vi "LEBITVacuum.ProcCases.vi"(0 "i ref in":refnum<vi>, 1 "selector":string, 2 "Data":T1, 3 "call cluster":T2={"Object"="", "Selector"="", "CallType"=enum."synchronous", "Async Object"="", "Async Selector"="", "Data Descriptor"="", "Data"=[], "Error #"=0, "Expire"=0}, 5 "error in (no error)":errorcluster) -> (14 "i ref out":refnum<vi>, 17 "answer cluster":T2={"Object"="", "Selector"="", "CallType"=enum."synchronous", "Async Object"="", "Async Selector"="", "Data Descriptor"="", "Data"=[], "Error #"=0, "Expire"=0}, 19 "error out":errorcluster)   [LabVIEW 2014, in "LEBITVacuum.lvlib"]
doc: "This method is called by a process from within the default case in the event loop. The methods of a class that are linked to events will be called from THIS method. Add your code here."
uses:
  LEBITVacuum.lvlib
  CS_Core/CSSystem/CoreDefs/CoreDefs.call_type.ctl
  CS_Core/BaseProcess/BaseProcess.descriptor string definition.ctl
  CS_Core/CSSystem/CoreDefs/CoreDefs.rawDataType.ctl
  CS_Core/CSSystem/CoreLib/CoreLib.byte array 2 short.vi
  CS_Core/CSSystem/CoreLib/CoreLib.string 2 byte array.vi
  CS_Core/CSSystem/CoreLib/CoreLib.byte array 2 string.vi
  CS_Core/BaseProcess/BaseProcess.lvlib
  CS_Core/CSSystem/CoreLib/CoreLib.lvlib
  CS_Core/CAEObj/CAEObj.lvlib
  CSlibraries-extern/DimLVEvent/LVDimInterface/LVDimInterface.lvlib
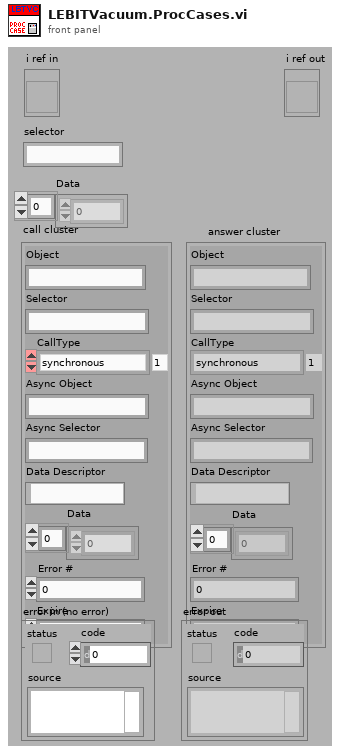
[diagram p1: front panel]
types:
  T1 = typedef "CoreDefs.rawDataType.ctl" = i8[]
  T2 = typedef "CoreDefs.call_type.ctl" = cluster{"Object":string, "Selector":string, "CallType":enum16{"simple", "synchronous", "asynchronous"}, "Async Object":string, "Async Selector":string, "Data Descriptor":T3, "Data":T1, "Error #":i32, "Expire":u32}
  T3 = typedef "BaseProcess.lvlib/BaseProcess.descriptor string definition.ctl" = string
  T4 = typedef "LEBITVacuum.lvlib/LEBITVacuum.i attribute.ctl" = cluster{"setValuePLC":string[], "nickNames":string[], "setValuePLCServiceID":i32[], "monValuePLC":string[], "SetValueServiceID":i32[], "MonValueServiceID":i32[], "SetValue":i16[], "AllPLCValues":string[], "CondSpecial2DArray":string[][], "CondSpecialIndex":i32[], "ReasonForLocking":string, "ReasonForLockingID":i32, "enableValuePLC":string[], "OverwriteCloseSafetyPLC":string[], "OverwriteOpenSafetyPLC":string[], "OverwriteCloseSafetyPLCServiceID":i32[], "OverwriteOpenSafetyPLCServiceID":i32[], "MKS Address Array":i32[][], "MKS MeasurementServiceID":i32[], "MKS Measurement":string[], "CRYO Measurement":string[][], "CRYO MeasurementServiceID":i32[], "Special":string[], "Start Date":string, "MKS VISA resource":refnum<visa-resource-name>, "CRYO VISA resource":refnum<visa-resource-name>}
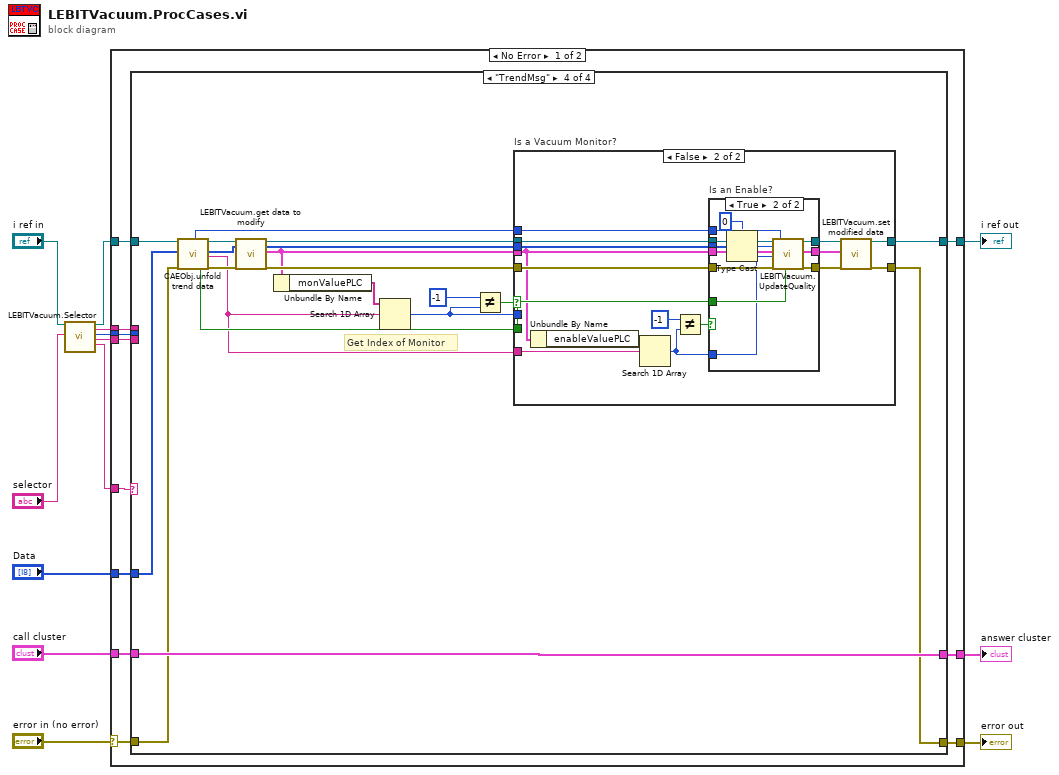
[diagram p0: block diagram]
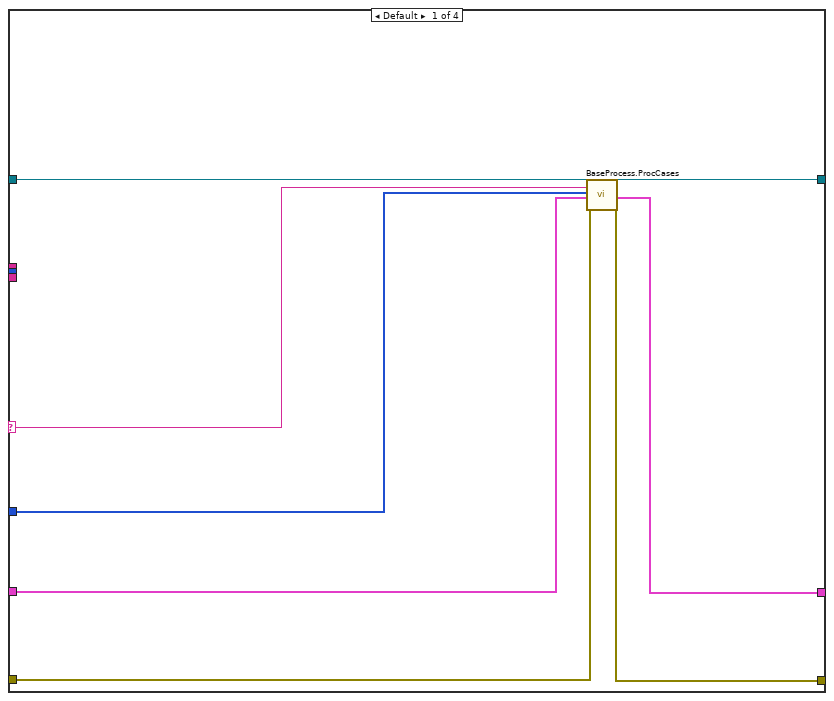
[diagram p2: hidden frame]
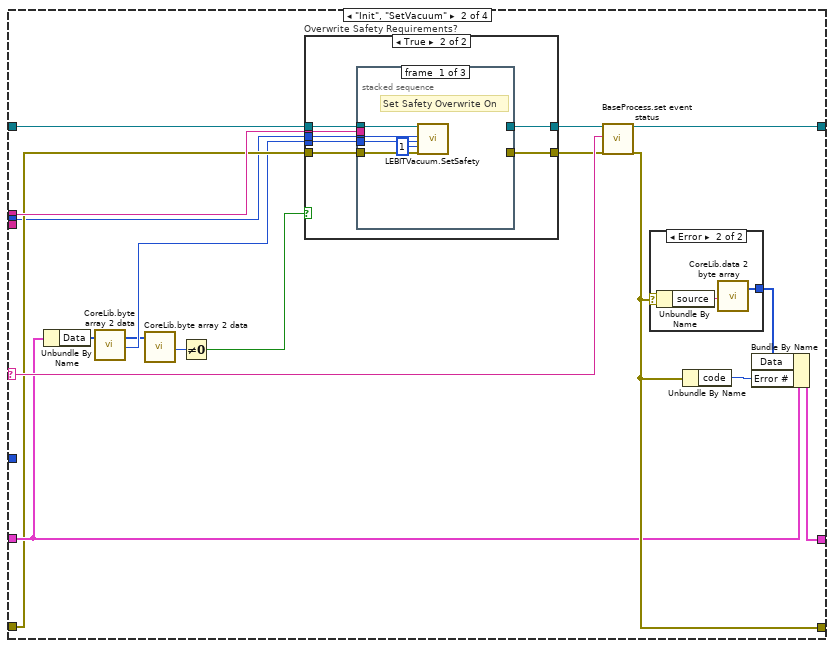
[diagram p3: hidden frame]
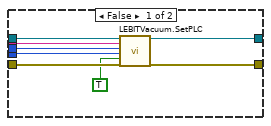
[diagram p4: hidden frame]
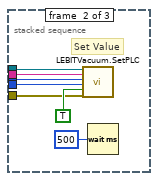
[diagram p5: hidden frame]
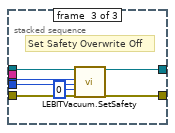
[diagram p6: hidden frame]
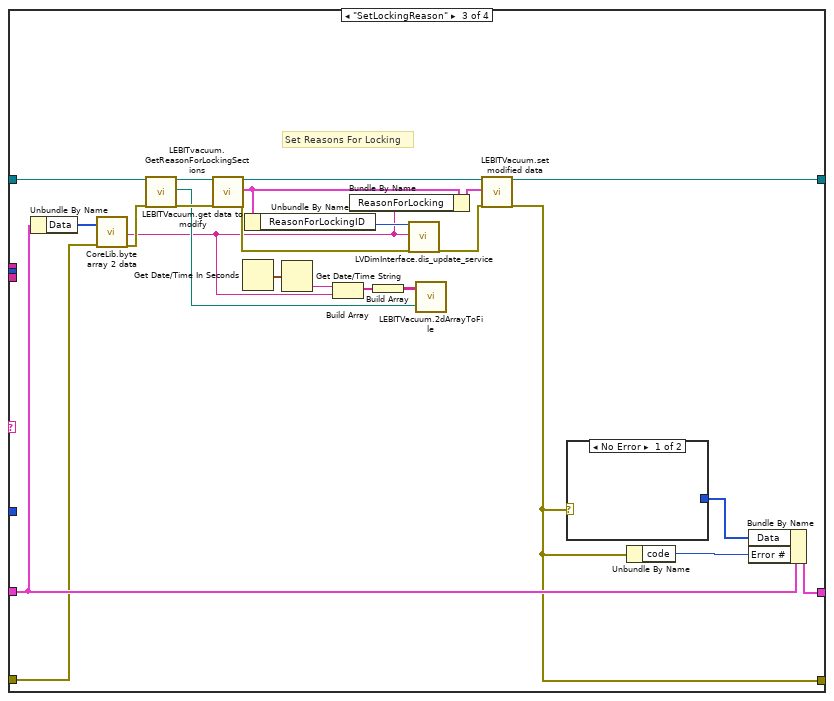
[diagram p8: hidden frame]
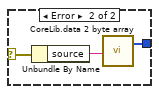
[diagram p9: hidden frame]
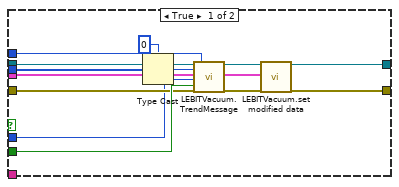
[diagram p10: hidden frame]
diagram:
  n1 = call "LEBITVacuum.Selector.vi"("i ref in"="i ref in", "selector in"="selector") -> ("i ref out"=w4:refnum<vi>, "Nickname"=w6:string, "index of element"=w3:i32, "Special Data"=w2:string, "selector out"=w7:string)  [unwired: 13 in]
  n2 = case shown="No Error" "error in (no error)" {
    selector: "error in (no error)" -> [w17 w179]
    tunnel: w7 -> [w24 _]
    tunnel: [w23 w180] -> w13
    tunnel: "Data" -> [w22 _]
    tunnel: "call cluster" -> [w21 w180]
    tunnel: w4 -> [w20 w181]
    tunnel: [w19 w181] -> w10
    tunnel: [w18 w179] -> w9
    tunnel: w6 -> [w16 _]
    tunnel: w3 -> [w15 _]
    tunnel: w2 -> [w14 _]
    frame No Error {
      n3 = case shown="\"TrendMsg\"" w24 {
        selector: w24 -> [w26 w45 _ _]
        tunnel: w22 -> [w27 _ _ w133]
        tunnel: w20 -> [w25 w39 w97 w132]
        tunnel: [w32 w46 w103 w115] -> w19
        tunnel: w21 -> [w28 w41 w108 w130]
        tunnel: [w29 w49 w106 w130] -> w23
        tunnel: w17 -> [w31 w38 w107 w129]
        tunnel: [w30 w47 w101 w116] -> w18
        tunnel: w16 -> [_ w42 _ _]
        tunnel: w15 -> [_ w36 _ _]
        tunnel: w14 -> [_ _ _ _]
        frame Default {
          # "In the default case, always call the ProcCase method of the parent class"
          n4 = call "BaseProcess.ProcCases.vi"("i ref in"=w25, "selector"=w26, "Data"=w27, "call cluster"=w28, "error in (no error)"=w31) -> ("i ref out"=w32:refnum<vi>, "answer cluster"=w29:T2, "error out"=w30:errorcluster)  [unwired: 12 in]
        }
        frame "Init", "SetVacuum" {
          n5 = Unbundle By Name(w41) -> ("Data"=w40:T1)
          n6 = call-poly "CoreLib.byte array 2 data.vi"("byteArray"=w40) -> ("byteArray out"=w35:T1, "i16"=w37:i16)  [unwired: 16 in, 1 out]
          n7 = call-poly "CoreLib.byte array 2 data.vi"("byteArray"=w35) -> ("i16"=w34:i16)  [unwired: 16 in, 2 out]
          n8 = Not Equal To 0?(x=w34) -> (x != 0?=w33:bool)
          n9 = case "Overwrite Safety Requirements?" shown="True" w33 {
            tunnel: [w58 w62] -> w44
            tunnel: [w57 w61] -> w43
            tunnel: w42 -> [w56 w59]
            tunnel: w39 -> [w55 w63]
            tunnel: w38 -> [w54 w65]
            tunnel: w37 -> [w52 w60]
            tunnel: w36 -> [w51 w64]
            frame False {
              n10 = call "LEBITVacuum.SetPLC.vi"("i ref in"=w55, "CommandName"=w56, "index of element"=w51, "Value"=w52, "log?"=TRUE, "error IO"=w54) -> ("i ref out"=w58:refnum<vi>, "error out"=w57:errorcluster)  [unwired: 12 in]
            }
            frame True {
              n11 = stacked-sequence {
                tunnel: w65 -> [w70 w73 w80]
                tunnel: w64 -> [w69 w75 w82]
                tunnel: w63 -> [w68 w76 w83]
                tunnel: [_ _ w79] -> w62
                tunnel: [_ _ w78] -> w61
                tunnel: w60 -> [w67 w74 w81]
                tunnel: w59 -> [_ w71 _]
                frame #0 {
                  # "Set Safety Overwrite On"
                  n12 = call "LEBITVacuum.SetSafety.vi"("i ref in"=w68, "index of element"=w69, "Set Value"=w67, "Safety Value"=i16 1, "error IO"=w70) -> ()  [unwired: 13 in, 2 out]
                }
                frame #1 {
                  # "Set Value"
                  n13 = call "LEBITVacuum.SetPLC.vi"("i ref in"=w76, "CommandName"=w71, "index of element"=w75, "Value"=w74, "log?"=TRUE, "error IO"=w73) -> ()  [unwired: 12 in, 2 out]
                  n14 = Wait (ms)(milliseconds to wait=u32 500) -> ()  [unwired: 1 out]
                }
                frame #2 {
                  # "Set Safety Overwrite Off"
                  n15 = call "LEBITVacuum.SetSafety.vi"("i ref in"=w83, "index of element"=w82, "Set Value"=w81, "Safety Value"=i16 0, "error IO"=w80) -> ("i ref out"=w79:refnum<vi>, "error out"=w78:errorcluster)  [unwired: 13 in]
                }
              }
            }
          }
          n16 = call "BaseProcess.set event status.vi"("i ref in"=w44, "EventStatus"=w45, "error in (no error)"=w43) -> ("i ref out"=w46:refnum<vi>, "error out"=w47:errorcluster)  [unwired: 14 in, 1 out]
          n17 = case shown="Error" w47 {
            selector: w47 -> [_ w87]
            tunnel: [_ w86] -> w48
            frame No Error {
            }
            frame Error {
              n18 = Unbundle By Name(w87) -> ("source"=w85:string)
              n19 = call-poly "CoreLib.data 2 byte array.vi"("string"=w85) -> ("byteArray out"=w86:T1)  [unwired: 18 in]
            }
          }
          n20 = Unbundle By Name(w47) -> ("code"=w50:i32)
          n21 = Bundle By Name(cluster=w41, "Data"=w48, "Error #"=w50) -> (w49:T2)
        }
        frame "SetLockingReason" {
          # "Set Reasons For Locking"
          n22 = Unbundle By Name(w108) -> ("Data"=w111:T1)
          n23 = call-poly "CoreLib.byte array 2 data.vi"("byteArray"=w111, "error in (no error)"=w107) -> ("string"=w90:string, "error out"=w94:errorcluster)  [unwired: 15 in, 1 out]
          n24 = call "LEBITvacuum.GetReasonForLockingSections.vi"("i ref in"=w97, "error in (no error)"=w94) -> ("i ref out"=w96:refnum<vi>, "Last Loaded File Loaction"=w93:path, "error out"=w95:errorcluster)  [unwired: 15 in]
          n25 = call "LEBITVacuum.get data to modify.vi"("i ref in"=w96, "error in (no error)"=w95) -> ("i ref out"=w102:refnum<vi>, "i attribute"=w100:T4, "error out"=w104:errorcluster)  [unwired: 14 in, 1 out]
          n26 = Get Date/Time In Seconds() -> (seconds since 1Jan1904=w92:timestamp)
          n27 = Unbundle By Name(w100) -> ("ReasonForLockingID"=w105:i32)
          n28 = Get Date/Time String(seconds (now)=w92) -> (time string=w91:string)  [unwired: 2 in, 1 out]
          n29 = Build Array(w91, w90) -> (w88:string[])
          n30 = Bundle By Name(cluster=w100, "ReasonForLocking"=w90) -> (w98:T4)
          n31 = Build Array(w88) -> (w89:string[][])
          n32 = call "LVDimInterface.dis_update_service.vi"("my_serviceID"=w105, "data"=w90, "error in (no error)"=w104) -> ("error out"=w99:errorcluster)  [unwired: 14 in, 2 out]
          n33 = call "LEBITVacuum.2dArrayToFile.vi"("file path (dialog if empty)"=w93, "Array"=w89) -> ()  [unwired: 2 in]
          n34 = call "LEBITVacuum.set modified data.vi"("i ref in"=w102, "i attribute"=w98, "error in (no error)"=w99) -> ("i ref out"=w103:refnum<vi>, "error out"=w101:errorcluster)  [unwired: 15 in]
          n35 = case shown="No Error" w101 {
            selector: w101 -> [_ w114]
            tunnel: [_ w113] -> w109
            frame No Error {
            }
            frame Error {
              n36 = Unbundle By Name(w114) -> ("source"=w112:string)
              n37 = call-poly "CoreLib.data 2 byte array.vi"("string"=w112) -> ("byteArray out"=w113:T1)  [unwired: 18 in]
            }
          }
          n38 = Unbundle By Name(w101) -> ("code"=w110:i32)
          n39 = Bundle By Name(cluster=w108, "Data"=w109, "Error #"=w110) -> (w106:T2)
        }
        frame "TrendMsg" {
          # "Get Index of Monitor"
          n40 = call "CAEObj.unfold trend data.vi"("i ref in"=w132, "raw trend data"=w133, "error in (no error)"=w129) -> ("quality"=w127:i32, "no link"=w120:bool, "i ref out"=w131:refnum<vi>, "data"=w123:i8[], "serviceName"=w119:string, "error out"=w128:errorcluster)  [unwired: 8 in, 3 out]
          n41 = call "LEBITVacuum.get data to modify.vi"("i ref in"=w131, "error in (no error)"=w128) -> ("i ref out"=w125:refnum<vi>, "i attribute"=w118:T4, "error out"=w126:errorcluster)  [unwired: 14 in, 1 out]
          n42 = Unbundle By Name(w118) -> ("monValuePLC"=w124:string[])
          n43 = Search 1D Array(1D array=w124, element=w119) -> (index of element=w117:i32)  [unwired: 1 in]
          n44 = Not Equal?(x=-1 ("y"), y=w117) -> (x != y?=w121:bool)
          n45 = case "Is a Vacuum Monitor?" shown="False" w121 {
            tunnel: w127 -> [w147 w163]
            tunnel: w120 -> [w146 w162]
            tunnel: w126 -> [w145 w161]
            tunnel: w125 -> [w144 w160]
            tunnel: w118 -> [w143 w156]
            tunnel: w123 -> [w142 w159]
            tunnel: [w138 w151] -> w115
            tunnel: [w137 w148] -> w116
            tunnel: w117 -> [w141 _]
            tunnel: w119 -> [_ w157]
            frame True {
              n46 = Type Cast(type=i16 0, x=w142) -> (*(type *) &x=w140:i16)
              n47 = call "LEBITVacuum.TrendMessage.vi"("i ref in"=w144, "data"=w140, "i attribute"=w143, "index"=w141, "error in"=w145, "quality"=w147, "no link"=w146) -> ("i ref out"=w136:refnum<vi>, "i attribute out"=w135:T4, "error out"=w134:errorcluster)  [unwired: 9 in, 1 out]
              n48 = call "LEBITVacuum.set modified data.vi"("i ref in"=w136, "i attribute"=w135, "error in (no error)"=w134) -> ("i ref out"=w138:refnum<vi>, "error out"=w137:errorcluster)  [unwired: 15 in]
            }
            frame False {
              n49 = Unbundle By Name(w156) -> ("enableValuePLC"=w158:string[])
              n50 = Search 1D Array(1D array=w158, element=w157) -> (index of element=w153:i32)  [unwired: 1 in]
              n51 = Not Equal?(x=-1 ("y"), y=w153) -> (x != y?=w154:bool)
              n52 = case "Is an Enable?" shown="True" w154 {
                tunnel: w163 -> [_ w178]
                tunnel: w162 -> [_ w177]
                tunnel: w161 -> [w164 w176]
                tunnel: w160 -> [w165 w175]
                tunnel: w159 -> [_ w172]
                tunnel: [w165 w171] -> w152
                tunnel: [w164 w170] -> w149
                tunnel: w153 -> [_ w169]
                tunnel: [w166 w168] -> w150
                tunnel: w156 -> [w166 w167]
                frame False {
                }
                frame True {
                  n53 = Type Cast(type=i16 0, x=w172) -> (*(type *) &x=w174:i16)
                  n54 = call "LEBITVacuum.UpdateQuality.vi"("i ref in"=w175, "data"=w174, "i attribute"=w167, "index"=w169, "error in"=w176, "quality"=w178, "no link"=w177) -> ("i ref out"=w171:refnum<vi>, "i attribute out"=w168:T4, "error out"=w170:errorcluster)  [unwired: 10 in]
                }
              }
              n55 = call "LEBITVacuum.set modified data.vi"("i ref in"=w152, "i attribute"=w150, "error in (no error)"=w149) -> ("i ref out"=w151:refnum<vi>, "error out"=w148:errorcluster)  [unwired: 15 in]
            }
          }
        }
      }
    }
    frame Error {
    }
  }
  "answer cluster" <- w13
  "i ref out" <- w10
  "error out" <- w9
